vi "SECoP_dataFindEnumerationValue.vi"(7 "Position":u32, 8 "error in (no error)":errorcluster, 9 "EnumName":string, 10 "SECoP_dataPtr":T1 {"ptr64" format="%.0x"; "ptr32" format="%.0x"}, 11 "DLL path (in)":T2) -> (0 "error out":errorcluster, 2 "EnumValue":i64, 3 "DLL path (out)":T2)   [LabVIEW 2015, in "SECoP.lvlib"]
doc: "Call <b>\"SECoP_dataFindEnumerationValue.vi\"</b> to access the integer value of an enumeration of a complex data type.\n\n<b>DLL path</b> input and output of cluster from \"SECoP-Initialize.vi\"\n<b>SECoP_dataPtr</b> data to access\n<b>Position</b> points to a virtual flattened entry of the data type; for a simple enumeration use 0\n<b>EnumName</b> name of the requested enumeration\n<b>EnumVal</b> enumeration value for the given name"
uses:
  SECoP.lvlib
  SECoP-data.ctl
  SECoP-libraries.ctl
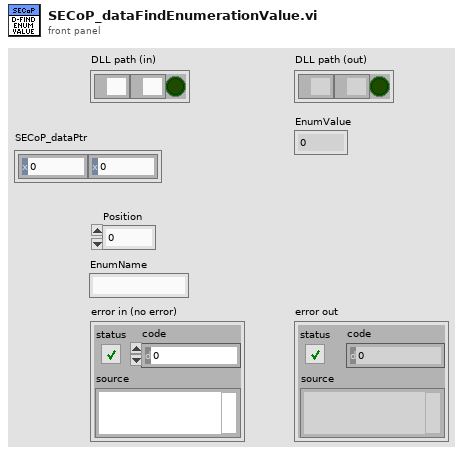
[diagram p1: front panel]
types:
  T1 = typedef "SECoP.lvlib/SECoP-data.ctl" = cluster{"ptr32":u32, "ptr64":u64}
  T2 = typedef "SECoP.lvlib/SECoP-libraries.ctl" = cluster{"serverDLL":path, "variantDLL":path, "cleanup_mode":bool}
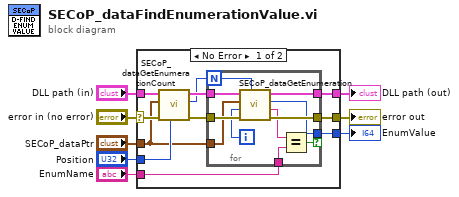
[diagram p0: block diagram]
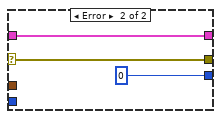
[diagram p2: hidden frame]
diagram:
  n1 = case shown="No Error" "error in (no error)" {
    selector: "error in (no error)" -> [w19 w32]
    tunnel: "DLL path (in)" -> [w18 w33]
    tunnel: [w11 w33] -> w3
    tunnel: [w10 w32] -> w2
    tunnel: "Position" -> [w14 _]
    tunnel: [w9 i64 0] -> w4
    tunnel: "SECoP_dataPtr" -> [w13 _]
    tunnel: "EnumName" -> [w12 _]
    frame No Error {
      n2 = call "SECoP_dataGetEnumerationCount.vi"("Position"=w14, "error in (no error)"=w19, "SECoP_dataPtr"=w13, "DLL path (in)"=w18) -> ("error out"=w16:errorcluster, "no. of enums"=w15:u32, "DLL path (out)"=w17:T2)  [unwired: 5 in]
      n3 = for {
        N: w15 -> [w28]
        tunnel: w17 -> [w30]
        tunnel: w16 -> [w29]
        tunnel: w13 -> [w27]
        tunnel: [w20] -> w9 if=w22
        tunnel: w12 -> [w23]
        tunnel: [w25] -> w11
        tunnel: [w24] -> w10
        i -> [w26]
        n4 = call "SECoP_dataGetEnumeration.vi"("Position"=w28, "error in (no error)"=w29, "Index"=w26, "SECoP_dataPtr in"=w27, "DLL path (in)"=w30) -> ("error out"=w24:errorcluster, "enumeration_name"=w21:string, "Enumval"=w20:i64, "DLL path (out)"=w25:T2)  [unwired: 3 in]
        n5 = Equal?(x=w21, y=w23) -> (x = y?=w22:bool)
      }
    }
    frame Error {
    }
  }
  "DLL path (out)" <- w3
  "error out" <- w2
  "EnumValue" <- w4
